vi "AutoGlobals.vi"() -> ()   [LabVIEW 2017]
panel:
  in  "AutonomousEnabled":bool
  in  "AutoFailed":bool
  out "EncoderRate":dbl
  in  "ZAxis":dbl
  in  "Speed":dbl
  in  "StrafeAngle":dbl
  out "CodeStatus":string
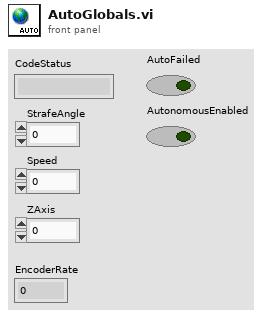
[diagram p1: front panel]
diagram:
